vi "ELVIS III v1.0 Write AO.vi"(7 "Scale Constants Array":T1, 8 "error in (no error)":errorcluster, 9 "dbl Scaled Value List":dbl[](array[numeric]), 10 "Channel List":T5, 11 "myRIO Ref In":T3) -> (0 "error out":errorcluster, 3 "myRIO Ref Out":T3)   [LabVIEW 2021]
uses:
  <vilib>/myRIO/Common/Instrument Driver Framework/myRIO v1.0/AO/typedefs/AO Channels List.ctl
  <vilib>/myRIO/Common/Instrument Driver Framework/myRIO v1.0/AO/typedefs/AO Channels Enum.ctl
  <vilib>/myRIO/Common/Instrument Driver Framework/Utilities/typedefs/myRIO v1.0 Reference.ctl
  <vilib>/myRIO/Common/Instrument Driver Framework/Utilities/typedefs/Generic FPGA Reference.ctl
  <vilib>/myRIO/Common/Instrument Driver Framework/Utilities/typedefs/Analog Scaling Constants List.ctl
  <vilib>/myRIO/Common/Instrument Driver Framework/Utilities/typedefs/Analog Scaling Constants.ctl
  <vilib>/myRIO/Common/Instrument Driver Framework/ELVIS III v1.0/AO/typedefs/ELVIS III AO Channels FPGA Reference.ctl
  <vilib>/rvi/errors/niLvFpgaAdjustHostInterfaceError.vi
  <vilib>/rvi/interface/nirviReadWriteControl/nirviReadWriteControl.xnode
  NiFpgaLv.dll
  <vilib>/rvi/interface/Simulation/niFpgaSimulationCallBeginRW.vi
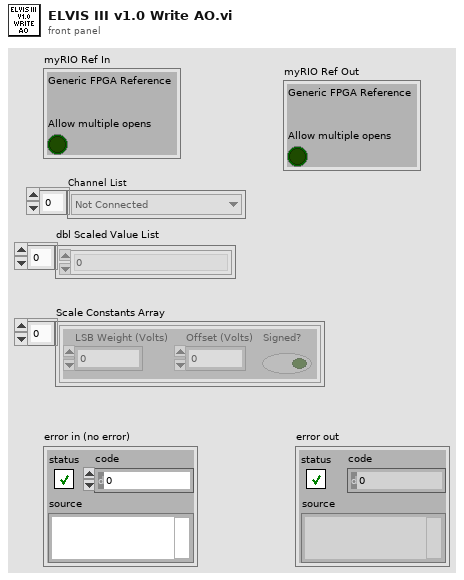
[diagram p1: front panel]
types:
  T1 = typedef "Analog Scaling Constants List.ctl" = T2[]
  T2 = typedef "Analog Scaling Constants.ctl" = cluster{"LSB Weight (Volts)":dbl, "Offset (Volts)":dbl, "Signed?":bool}
  T3 = typedef "myRIO v1.0 Reference.ctl" = cluster{"Generic FPGA Reference":T4, "Allow multiple opens":bool}
  T4 = typedef "Generic FPGA Reference.ctl" = refnum<k20>
  T5 = typedef "AO Channels List.ctl" = T6[]
  T6 = typedef "AO Channels Enum.ctl" = enum16{"Not Connected", "AudioOut/Left", "AudioOut/Right", "C/AO0", "C/AO1", "A/AO0", "A/AO1", "B/AO0", "B/AO1"}
  T7 = typedef "ELVIS III AO Channels FPGA Reference.ctl" = refnum<k20>
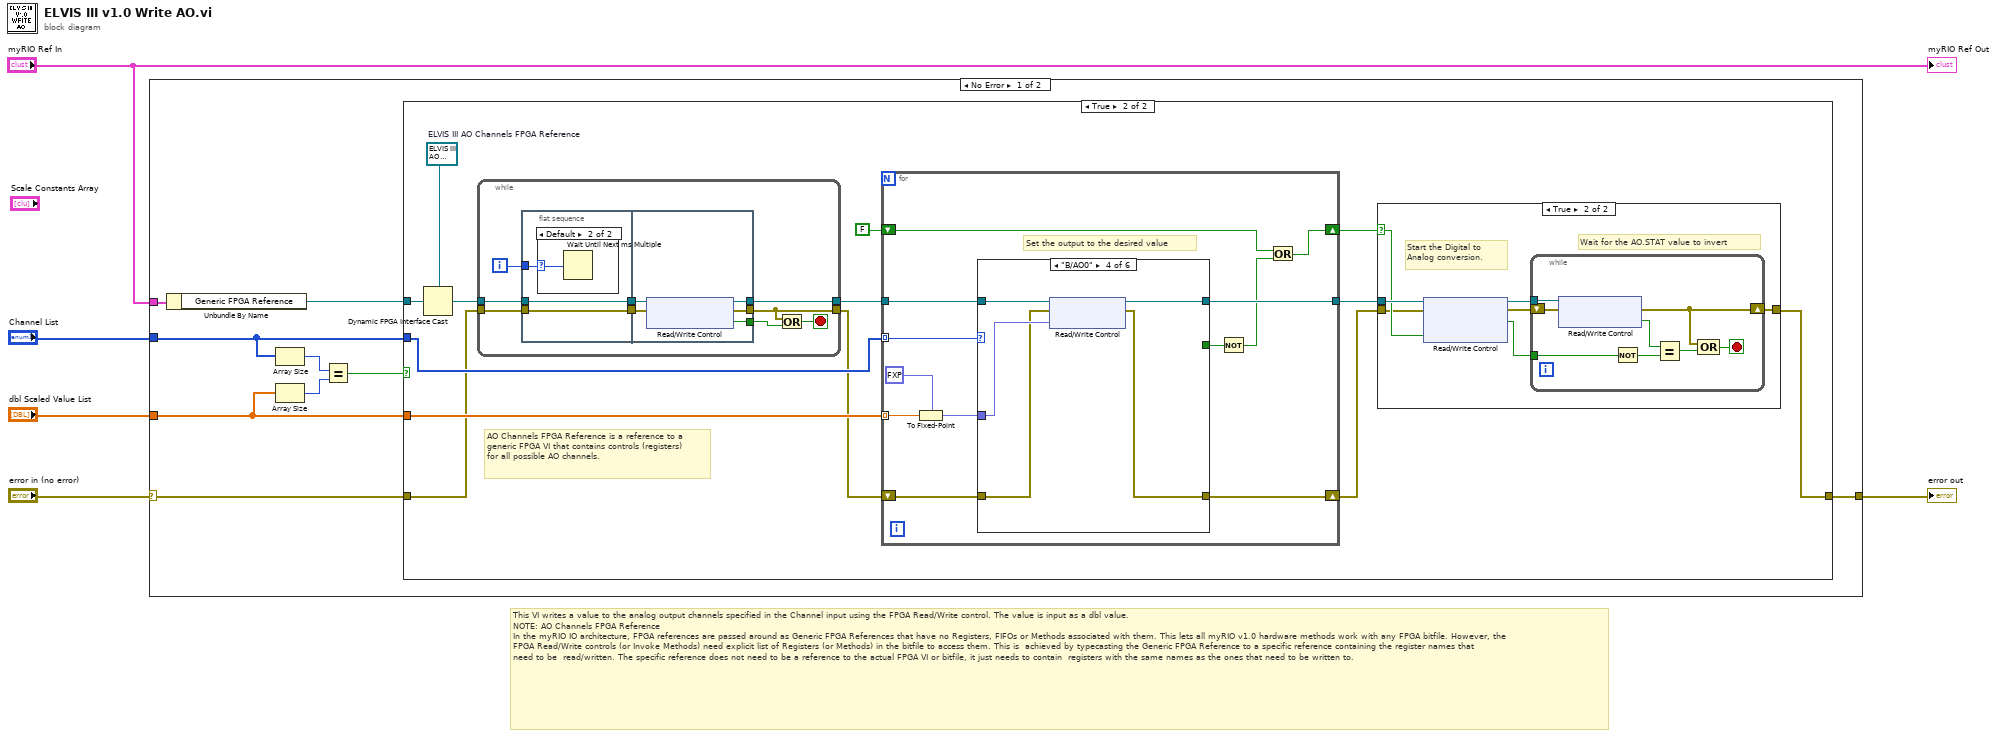
[diagram p0: block diagram]
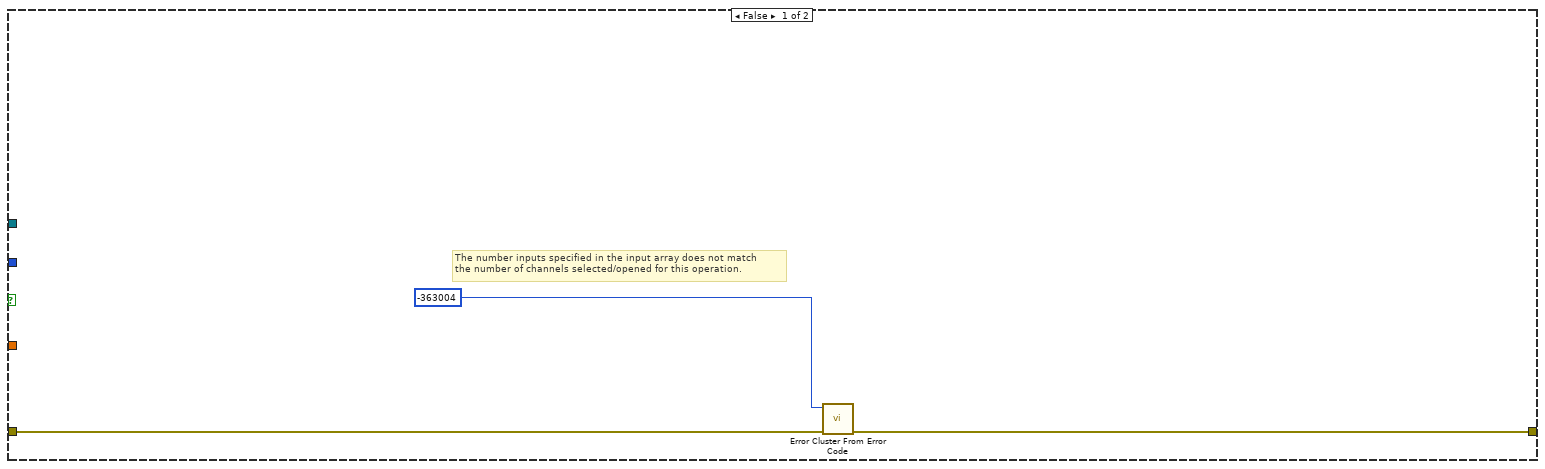
[diagram p2: hidden frame]
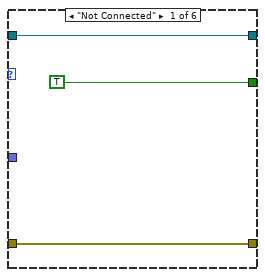
[diagram p5: hidden frame]
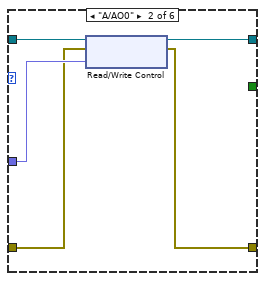
[diagram p6: hidden frame]
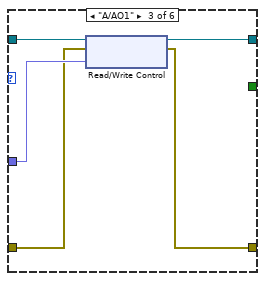
[diagram p7: hidden frame]
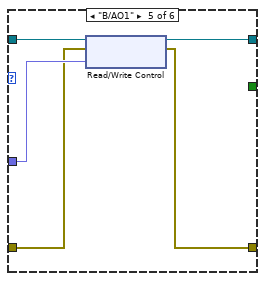
[diagram p8: hidden frame]
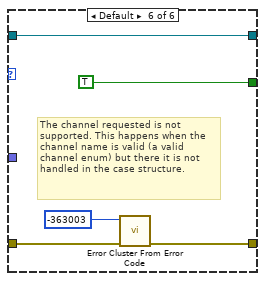
[diagram p9: hidden frame]
diagram:
  # "This VI writes a value to the analog output channels specified in the Channel input using the FPGA Read/Write control. The value is input as a dbl value.\nNOTE: AO Channels FPGA Reference\nIn the myRIO IO architecture, FPGA references are passed around as Generic FPGA References that have no Registers, FIFOs or Methods associated with them. This lets all myRIO v1.0 hardware methods work with any FPGA bitfile. However, the  FPGA Read/Write controls (or Invoke Methods) need explicit list of Registers (or Methods) in the bitfile to access them. This is  achieved by typecasting the Generic FPGA Reference to a specific reference containing the register names that need to be  read/written. The specific reference does not need to be a reference to the actual FPGA VI or bitfile, it just needs to contain  registers with the same names as the ones that need to be written to."
  n1 = case shown="No Error" "error in (no error)" {
    selector: "error in (no error)" -> [w10 w105]
    tunnel: [w14 w105] -> w5
    tunnel: "Channel List" -> [w13 _]
    tunnel: "dbl Scaled Value List" -> [w12 _]
    tunnel: "myRIO Ref In" -> [w9 _]
    frame No Error {
      n2 = Unbundle By Name(w9) -> ("Generic FPGA Reference"=w8:T4)
      n3 = Array Size(array=w12) -> (size(s)=w11:i32)
      n4 = Array Size(array=w13) -> (size(s)=w7:i32)
      n5 = Equal?(x=w7, y=w11) -> (x = y?=w6:bool)
      n6 = case shown="True" w6 {
        tunnel: w10 -> [w17 w19]
        tunnel: w8 -> [_ w27]
        tunnel: [w16 w22] -> w14
        tunnel: w13 -> [_ w29]
        tunnel: w12 -> [_ w28]
        frame False {
          # "The number inputs specified in the input array does not match\nthe number of channels selected/opened for this operation."
          n7 = call <vilib>:"Error Cluster From Error Code.vi"("error in (no error)"=w17, "error code (0)"=-363004) -> ("error out"=w16:errorcluster)  [unwired: 7 in]
        }
        frame True {
          w30 = T7 refnum  # ELVIS III AO Channels FPGA Reference
          # "AO Channels FPGA Reference is a reference to a generic FPGA VI that contains controls (registers) for all possible AO channels."
          n8 = Dynamic FPGA Interface Cast(Session In=w30, Type=w27) -> (Session Out=w21:T7)
          n9 = while {
            tunnel: w21 -> [w39]
            tunnel: w19 -> [w38]
            tunnel: [w35] -> w18
            tunnel: [w32] -> w20
            i -> [w31]
            stop <- w33 stop-if-true
            n10 = flat-sequence {
              tunnel: w38 -> [w41]
              tunnel: w39 -> [w42]
              tunnel: [w42] -> w37
              tunnel: [w41] -> w36
              tunnel: w31 -> [w40]
              tunnel: [w46] -> w34
              tunnel: [w45] -> w35
              tunnel: w37 -> [w48]
              tunnel: w36 -> [w47]
              tunnel: [w44] -> w32
              frame #0 {
                n11 = case shown="Default" w40 {
                  selector: w40 -> [_ w43]
                  frame 0 {
                  }
                  frame Default {
                    n12 = Wait Until Next ms Multiple(millisecond multiple=w43) -> ()  [unwired: 1 out]
                  }
                }
              }
              frame #1 {
                n13 = xnode "Read/Write Control"("FPGA VI Reference In"=w48, "error in"=w47) -> ("FPGA VI Reference Out"=w44:T7, "error out"=w45:errorcluster, "DMA.SYS.RDY"=w46:bool)
              }
            }
            n14 = Or(x=w35, y=w34) -> (x .or. y?=w33:bool)
          }
          n15 = for {
            tunnel: w20 -> [w76]
            tunnel: w28 -> [w67] mode=indexing
            tunnel: w29 -> [w73] mode=indexing
            shift-right: [w74] -> w25
            shift-left: w18 -> [w75]
            tunnel: [w72] -> w26
            shift-right: [w71] -> w23
            shift-left: FALSE ("AO.GO") -> [w70]
            # "Set the output to the desired value"
            n16 = To Fixed-Point(fixed-point type=fxp<+/-,20,5> 0.0, number=w67) -> (fixed-point=w66:fxp<+/-,20,5>)
            n17 = case shown="\"B/AO0\"" w73 {
              tunnel: w75 -> [w79 w80 w85 w90 w95 w102]
              tunnel: [w79 w81 w86 w91 w96 w103] -> w74
              tunnel: w76 -> [w78 w84 w89 w94 w99 w101]
              tunnel: [w78 w83 w88 w93 w98 w101] -> w72
              tunnel: [TRUE ("AO.GO") _ _ _ _ TRUE ("AO.GO")] -> w69
              tunnel: w66 -> [_ w82 w87 w92 w97 _]
              frame "Not Connected" {
              }
              frame "A/AO0" {
                n18 = xnode "Read/Write Control"("FPGA VI Reference In"=w84, "error in"=w80, "AO.A_0.VAL"=w82) -> ("FPGA VI Reference Out"=w83:T7, "error out"=w81:errorcluster)
              }
              frame "A/AO1" {
                n19 = xnode "Read/Write Control"("FPGA VI Reference In"=w89, "error in"=w85, "AO.A_1.VAL"=w87) -> ("FPGA VI Reference Out"=w88:T7, "error out"=w86:errorcluster)
              }
              frame "B/AO0" {
                n20 = xnode "Read/Write Control"("FPGA VI Reference In"=w94, "error in"=w90, "AO.B_0.VAL"=w92) -> ("FPGA VI Reference Out"=w93:T7, "error out"=w91:errorcluster)
              }
              frame "B/AO1" {
                n21 = xnode "Read/Write Control"("FPGA VI Reference In"=w99, "error in"=w95, "AO.B_1.VAL"=w97) -> ("FPGA VI Reference Out"=w98:T7, "error out"=w96:errorcluster)
              }
              frame Default {
                # "The channel requested is not supported. This happens when the channel name is valid (a valid channel enum) but there it is not handled in the case structure."
                n22 = call <vilib>:"Error Cluster From Error Code.vi"("error in (no error)"=w102, "error code (0)"=-363003) -> ("error out"=w103:errorcluster)  [unwired: 7 in]
              }
            }
            n23 = Not(x=w69) -> (.not. x?=w68:bool)
            n24 = Or(x=w70, y=w68) -> (x .or. y?=w71:bool)
          }
          n25 = case shown="True" w23 {
            selector: w23 -> [_ w55]
            tunnel: w26 -> [_ w56]
            tunnel: w25 -> [w49 w54]
            tunnel: [w49 w50] -> w22
            frame False {
            }
            frame True {
              # "Wait for the AO.STAT value to invert"
              # "Start the Digital to Analog conversion."
              n26 = xnode "Read/Write Control"("FPGA VI Reference In"=w56, "error in"=w54, "AO.SYS.GO"=w55) -> ("FPGA VI Reference Out"=w53:T7, "error out"=w52:errorcluster, "AO.SYS.STAT"=w51:bool)
              n27 = while {
                tunnel: w51 -> [w61]
                tunnel: w53 -> [w63]
                shift-right: [w58] -> w50
                shift-left: w52 -> [w64]
                stop <- w59 stop-if-true
                n28 = xnode "Read/Write Control"("FPGA VI Reference In"=w63, "error in"=w64) -> ("error out"=w58:errorcluster, "AO.SYS.STAT"=w62:bool)  [unwired: 1 out]
                n29 = Not(x=w61) -> (.not. x?=w60:bool)
                n30 = Equal?(x=w62, y=w60) -> (x = y?=w57:bool)
                n31 = Compound Arithmetic op=OR(w58, w57) -> (w59:bool)
              }
            }
          }
        }
      }
    }
    frame Error {
      # "There is an incoming error so there is nothing to do."
    }
  }
  "error out" <- w5
  "myRIO Ref Out" <- "myRIO Ref In"
